vi "Solve2.vi"(8 "Error In":errorcluster, 11 "object in":refnum<class "2022_3.lvclass">) -> (0 "Error Out":errorcluster, 2 "Result":u64, 3 "object out":refnum<class "2022_3.lvclass">)   [LabVIEW 2020, in "2022_3.lvclass"]
uses:
  2022_3.lvclass
  2022_3.lvclass/2022_3.ctl
  e5e0ac7a-7674-4fae-a817-b3bd16ac171a.vi
  472c50c8-ce80-4600-aecc-683402f0aa07.vi
  bee7fda4-5776-47a9-a5c6-27aa94bd60ca.vi
  e5e0ac7a-7674-4fae-a817-b3bd16ac171a.vi/be6f088c-3e4b-4523-ad48-2cdc85bad38a.vi
  e5e0ac7a-7674-4fae-a817-b3bd16ac171a.vi/f202eadf-433e-4cdb-b986-b2351ce8d73c.vi
  e5e0ac7a-7674-4fae-a817-b3bd16ac171a.vi/094751bc-bcf2-4346-afae-53942128b536.vi
  e5e0ac7a-7674-4fae-a817-b3bd16ac171a.vi/06ee343e-764f-4086-89d5-f578778d243c.vi
panel:
  out "Letter":string
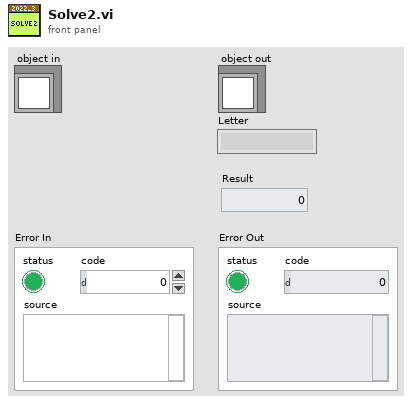
[diagram p1: front panel]
types:
  T1 = cluster{"Compartment1":u8[], "Compartment2":u8[]}[]
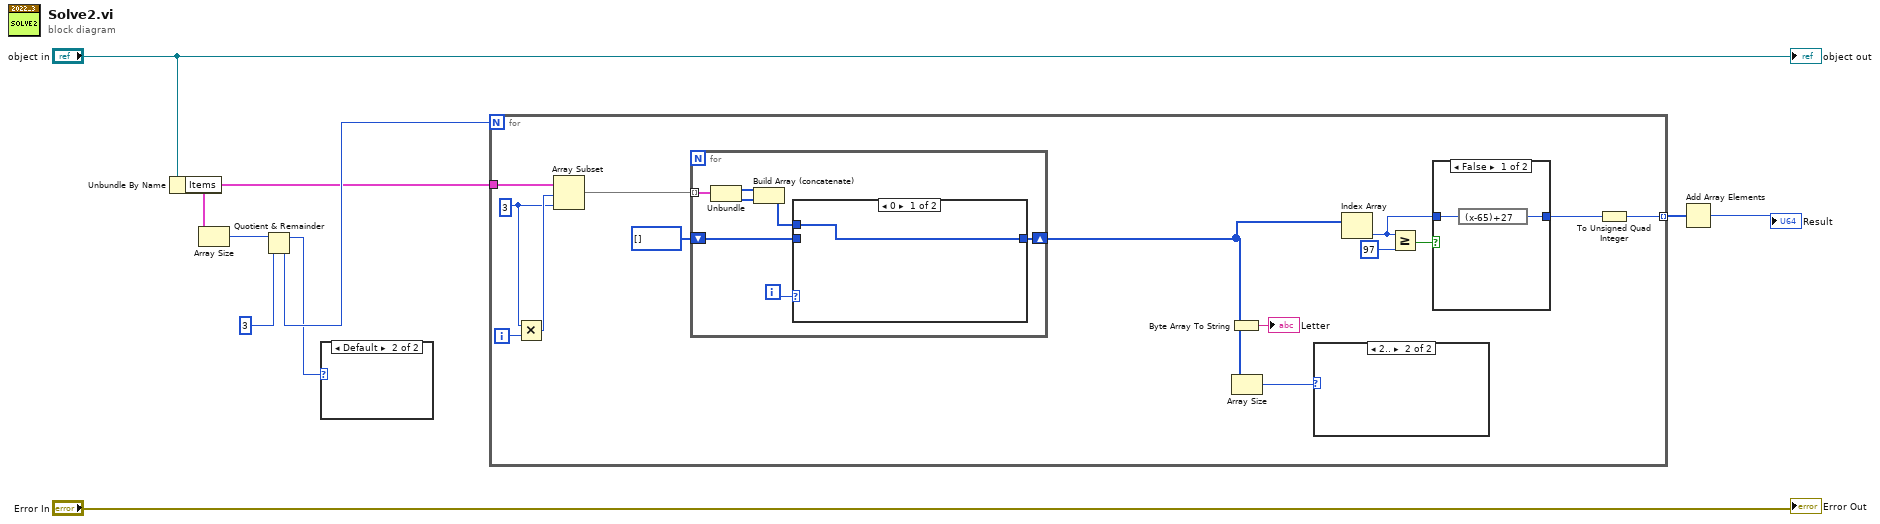
[diagram p0: block diagram]
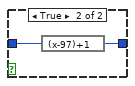
[diagram p3: hidden frame]
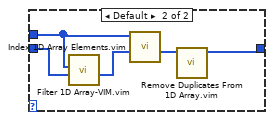
[diagram p5: hidden frame]
diagram:
  n1 = Unbundle By Name("object in") -> ("Items"=w3:T1)
  n2 = Array Size(array=w3) -> (size(s)=w7:i32)
  n3 = Quotient & Remainder(x=w7, y=3) -> (x-y*floor(x/y)=w4:i32, floor(x/y)=w5:i32)
  n4 = case shown="Default" w4 {
    frame 0 {
    }
    frame Default {
    }
  }
  n5 = for {
    N: w5 -> [_]
    tunnel: w3 -> [w23]
    tunnel: [w10] -> w2 mode=indexing
    i -> [w22]
    w20 = 3 ("y")
    n6 = Multiply(x=w20, y=w22) -> (x*y=w21:i32)
    n7 = Array Subset(array=w23, index=w21, length=w20) -> (w19:T1)
    n8 = for {
      tunnel: w19 -> [w34] mode=indexing
      shift-right: [w29] -> w11
      shift-left: u8[] [] ("array with duplicates removed") -> [w28]
      i -> [w31]
      n9 = Unbundle(w34) -> ("Compartment1"=w33:u8[], "Compartment2"=w32:u8[])
      n10 = Build Array (concatenate)(w33, w32) -> (w30:u8[])
      n11 = case shown="0" w31 {
        tunnel: w30 -> [w35 w38]
        tunnel: [w35 w36] -> w29
        tunnel: w28 -> [_ w37]
        frame 0 {
        }
        frame Default {
          n12 = call "Filter 1D Array-VIM.vim"("Item(s) to Filter"=w37, "Array"=w38) -> ("Filtered Item Indices"=w40:i32[])  [unwired: 5 in, 1 out]
          n13 = call "Index 1D Array Elements.vim"("indices"=w40, "array"=w38) -> ("elements"=w39:u8[])  [unwired: 9 in]
          n14 = call "Remove Duplicates From 1D Array.vim"("array"=w39) -> ("array with duplicates removed"=w36:u8[])  [unwired: 10 in]
        }
      }
    }
    n15 = Byte Array To String(unsigned byte array=w11) -> (string=→"Letter":string)
    n16 = Array Size(array=w11) -> (size(s)=w17:i32)
    n17 = case shown="2.." w17 {
      frame 0, Default {
      }
      frame 2.. {
      }
    }
    n18 = Index Array(array=w11) -> (element=w14:u8)  [unwired: 1 in]
    n19 = Greater Or Equal?(x=w14, y=u8 97) -> (x >= y?=w13:bool)
    n20 = case shown="False" w13 {
      tunnel: w14 -> [w25 w27]
      tunnel: [w24 w26] -> w15
      frame False {
        n21 = expression code="(x-65)+27"(w25) -> (w24:u8)
      }
      frame True {
        n22 = expression code="(x-97)+1"(w27) -> (w26:u8)
      }
    }
    n23 = To Unsigned Quad Integer(1:w15) -> (0:w10:u64)
  }
  n24 = Add Array Elements(numeric array=w2) -> (sum=→"Result":u64)
  "Error Out" <- "Error In"
  "object out" <- "object in"
